vi "Histogram2DManual1001.vi"   [LabVIEW 2013]
uses:
  <vilib>/Heliosphere Research LLC/Advanced Plotting Toolkit/api_plotting/Histogram2DProperties.ctl
  <vilib>/Heliosphere Research LLC/Advanced Plotting Toolkit/properties/Colormap.ctl
  <vilib>/Heliosphere Research LLC/Advanced Plotting Toolkit/properties/Colormap_Map.ctl
  <vilib>/Heliosphere Research LLC/Advanced Plotting Toolkit/properties/Colormap_Scaling.ctl
  <vilib>/Heliosphere Research LLC/Advanced Plotting Toolkit/properties/Display.ctl
  <vilib>/Heliosphere Research LLC/Advanced Plotting Toolkit/api_plotting/Histogram2D_Manual.vi
  <vilib>/Heliosphere Research LLC/Advanced Plotting Toolkit/Advanced Plotting Toolkit.lvlib
types:
  T1 = typedef "Advanced Plotting Toolkit.lvlib/Colormap_Map.ctl" = enum16{"Automatic", "Rainbow", "Hot and Cold", "White-Black", "White-Blue", "White-Green", "White-Red", "Fire", "Water", "Earth", "Air", "Pastel", "Banded", "Stepped"}
  T2 = typedef "Advanced Plotting Toolkit.lvlib/Histogram2DProperties.ctl" = cluster{"Normalize":bool, "Colormap":T3, "Display":T5}
  T3 = typedef "Advanced Plotting Toolkit.lvlib/Colormap.ctl" = cluster{"Map":T1, "Value Min":dbl, "Value Max":dbl, "Scaling":T4, "Reverse":bool}
  T4 = typedef "Advanced Plotting Toolkit.lvlib/Colormap_Scaling.ctl" = enum16{"Default"}
  T5 = typedef "Advanced Plotting Toolkit.lvlib/Display.ctl" = cluster{"Alpha":dbl, "Z Order":dbl}
  T6 = typedef "Advanced Plotting Toolkit.lvlib/PlotID.ctl" = i32
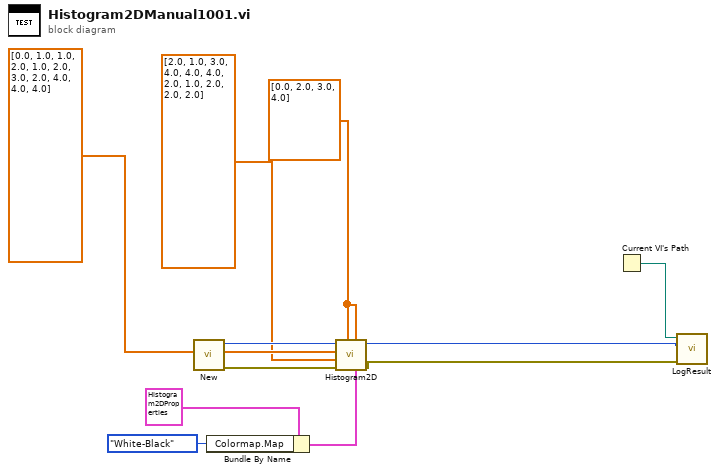
[diagram p0: block diagram]
diagram:
  w1 = dbl[] [0.0, 2.0, 3.0, 4.0] ("X Bin Edges")
  n1 = call <vilib>:"New.vi"() -> ("error out"=w9:errorcluster, "Plot ID"=w10:T6)  [unwired: 10 in]
  n2 = Bundle By Name(cluster=T2 {"Normalize"=FALSE, "Colormap"={"Map"=enum."Automatic", "Value Min"=nan, "Value Max"=nan, "Scaling"=enum."Default", "Reverse"=FALSE}, "Display"={"Alpha"=nan, "Z Order"=nan}} ("Histogram 2D Properties"), "Colormap.Map"=Colormap_Map."White-Black") -> (w5:T2)
  n3 = call-poly <vilib>:"Histogram2D.vi"("Properties"=w5, "Y Bin Edges"=w1, "X Bin Edges"=w1, "error in (no error)"=w9, "Y Data"=dbl[] [2.0, 1.0, 3.0, 4.0, 4.0, 4.0, 2.0, 1.0, 2.0, 2.0, 2.0] ("X Data"), "X Data"=dbl[] [0.0, 1.0, 1.0, 2.0, 1.0, 2.0, 3.0, 2.0, 4.0, 4.0, 4.0], "Plot ID"=w10) -> ("error out"=w3:errorcluster, "Plot ID Out"=w4:T6)  [unwired: 3 in]
  n4 = Current VI's Path() -> (path=w11:path)
  n5 = call "LogResult.vi"("Test Result"=w3, "Test Artifact"=w4, "VI Path"=w11) -> ()  [unwired: 9 in]
